vi "To File.vi"   [LabVIEW 2016, in "JSON Value.lvclass"]
doc: "Saves a JSON instance's data to the given file."
uses:
  JSON Value.lvclass
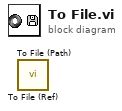
[diagram p0: block diagram]
diagram:
  n1 = call "To File (Ref).vi"() -> ()  [unwired: 10 in, 2 out]
  n2 = call "To File (Path).vi"() -> ()  [unwired: 11 in, 1 out]
